vi "Test Report Contain TestCase Segment.vi"(8 "error in (no error)":errorcluster, 11 "XML Report Test in":refnum<class "XML Report Test.lvclass">) -> (0 "error out":errorcluster, 3 "XML Report Test out":refnum<class "XML Report Test.lvclass">)   [LabVIEW 2020, in "XML Report Test.lvclass"]
uses:
  XML Report Test.lvclass
  XML Report Test.lvclass/XML Report Test.ctl
  source/Plugins/XML Report/XML Report.lvclass
panel:
  out "Report Content":string
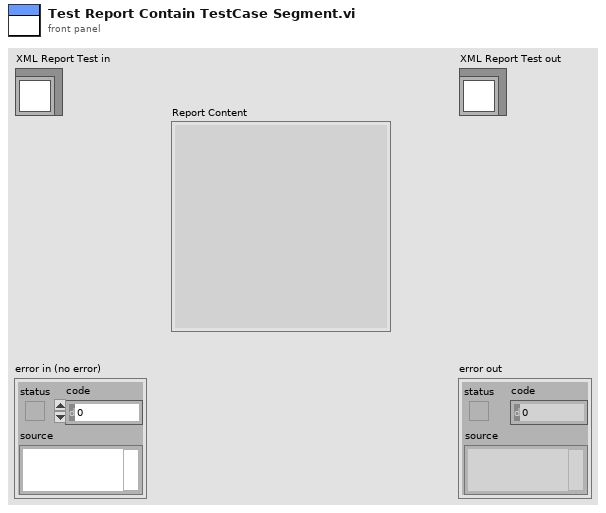
[diagram p1: front panel]
types:
  T1 = typedef "Result.lvlib/Result.ctl" = cluster{"Name":string, "Description":string, "Status":T2, "Result Type":T3, "Execution Time":dbl, "Data":cluster{"Expected":variant, "Actual":variant, "Delta":variant}}
  T2 = typedef "Result.lvlib/Status.ctl" = enum16{"", "Passed", "Failed", "Error", "Skipped", "Setup Error", "Broken", "Teardown Error"}
  T3 = typedef "Result.lvlib/Type.ctl" = enum16{"Test Case", "Test Suite", "Test Run", "Pass", "Fail", "Skip", "Pass if", "Fail if", "Pass if Error", "Fail if Error", "Pass if Equal", "Fail if Equal"}
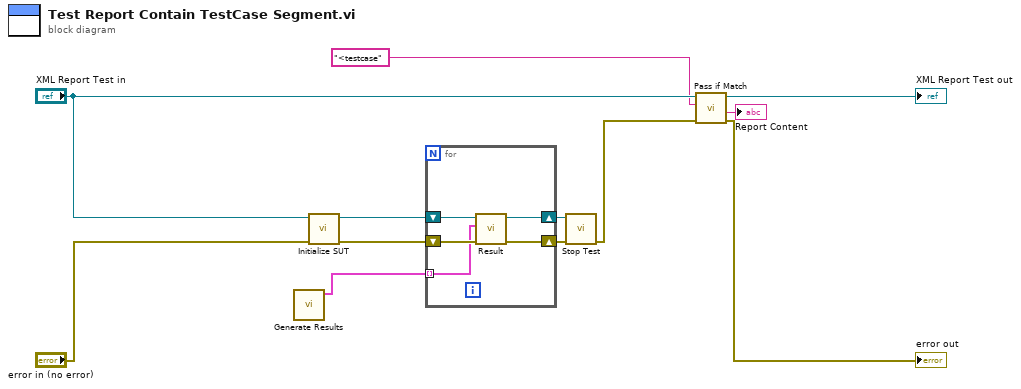
[diagram p0: block diagram]
diagram:
  n1 = call "Generate Results.vi"() -> ("Data"=w4:T1[])  [unwired: 10 in, 1 out]
  n2 = call "Initialize SUT.vi"("error in (no error)"="error in (no error)", "XML Report Test in"="XML Report Test in") -> ("error out"=w2:errorcluster, "XML Report out"=w1:refnum<class "XML Report.lvclass">)  [unwired: 8 in]
  n3 = for {
    shift-right: [w16] -> w6
    shift-left: w2 -> [w17]
    shift-right: [w14] -> w5
    shift-left: w1 -> [w15]
    tunnel: w4 -> [w13] mode=indexing
    n4 = call-dynamic "Result.vi"("error in (no error)"=w17, "Result"=w13, "XML Report In"=w15) -> ("error out"=w16:errorcluster, "XML Report Out"=w14:refnum<class "XML Report.lvclass">)  [unwired: 7 in]
  }
  n5 = call-dynamic "Stop Test.vi"("error in (no error)"=w6, "XML Report In"=w5) -> ("error out"=w9:errorcluster)  [unwired: 8 in, 1 out]
  n6 = call "Pass if Match.vi"("error in (no error)"=w9, "regular expression"="<testcase", "XML Report Test in"="XML Report Test in") -> ("error out"=→"error out":errorcluster, "Report Content"=→"Report Content":string, "XML Report Test out"=→"XML Report Test out":refnum<class "XML Report Test.lvclass">)  [unwired: 6 in]
